vi "Set Drop Down Width.vi"(8 "error in":errorcluster, 10 "Drop Down Width":i32, 11 "Combo Box in":refnum<class "Combo Box.lvclass">) -> (0 "error out":errorcluster, 3 "Combo Box out":refnum<class "Combo Box.lvclass">)   [LabVIEW 2023, in "SourceGrid.lvlib" / "Combo Box.lvclass"]
uses:
  Combo Box.lvclass
  Combo Box.lvclass/Combo Box.ctl
  D:/git/Sourcegrid-LabVIEW/dll/SourceGrid.dll
  dll/SourceGrid.dll
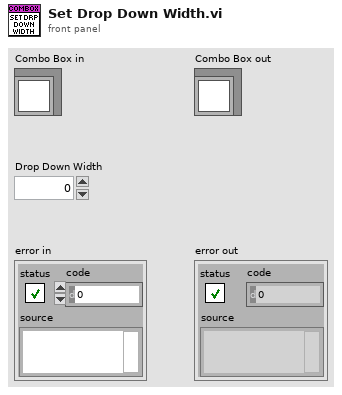
[diagram p1: front panel]
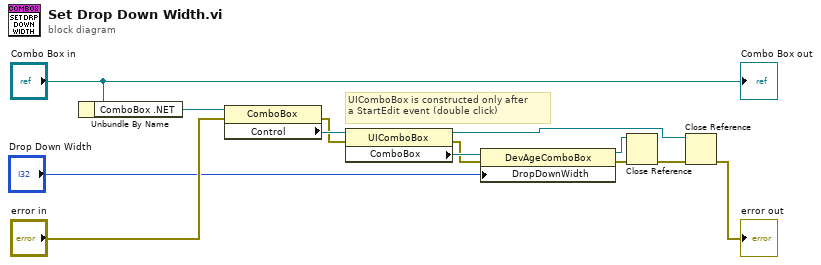
[diagram p0: block diagram]
diagram:
  # "UIComboBox is constructed only after\na StartEdit event (double click)"
  n1 = Unbundle By Name("Combo Box in") -> ("ComboBox .NET"=w12:refnum<k24>)
  n2 = property class="ComboBox"(reference=w12, error in="error in") -> (error out=w7:errorcluster, "Control"=w10:refnum<k24>)  [unwired: 1 out]
  n3 = property class="UIComboBox"(reference=w10, error in=w7) -> (reference out=w1:refnum<k24>, error out=w6:errorcluster, "ComboBox"=w9:refnum<k24>)
  n4 = property class="DevAgeComboBox"(reference=w9, error in=w6, "DropDownWidth"="Drop Down Width") -> (reference out=w3:refnum<k24>, error out=w5:errorcluster)
  n5 = Close Reference(reference=w3, error in (no error)=w5) -> (error out=w4:errorcluster)
  n6 = Close Reference(reference=w1, error in (no error)=w4) -> (error out=→"error out":errorcluster)
  "Combo Box out" <- "Combo Box in"
